vi "ArraysFunctionswithLoops.vi"() -> ()   [LabVIEW 2020]
panel:
  out "Array":i32[][](array[numeric])
  out "Numeric":i32
  in  "stop":bool
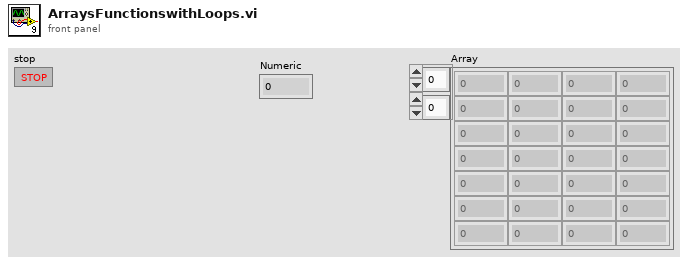
[diagram p1: front panel]
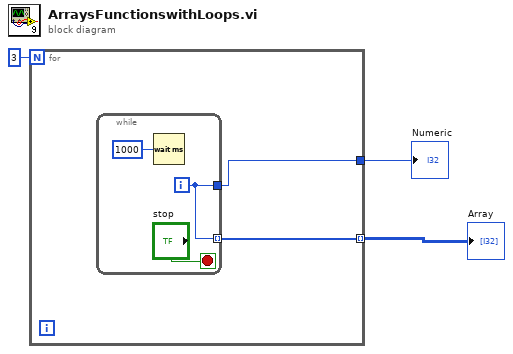
[diagram p0: block diagram]
diagram:
  n1 = for {
    N: 3 -> [_]
    tunnel: [w5] -> w2
    tunnel: [w4] -> w1 mode=indexing
    n2 = while {
      tunnel: [w7] -> w4 mode=indexing
      tunnel: [w7] -> w5
      i -> [w7]
      stop <- "stop" stop-if-true
      n3 = Wait (ms)(milliseconds to wait=u32 1000) -> ()  [unwired: 1 out]
    }
  }
  "Numeric" <- w2
  "Array" <- w1
